vi "SVPO Analog Tacho Process (N Ch DBL WDT).vi"(0 "analog tacho signal":waveform(dbl)={"t0"=timestamp(0 s since 1904-01-01), "dt"=0.0, "Y"=[]}, 1 "AnalogTach States":T1, 5 "PPR":dbl, 7 "Thresh(V)":dbl, 9 "Slope":u16, 11 "hysteresis (0)":dbl format="%.2f", 12 "pulse width (2)":i32=2) -> (3 "AnalogTach States Out":T1, 4 "speed position info":T2)   [LabVIEW 2018, in "Measurement Channels.lvlib" / "Tachometer.lvclass"]
doc: "Locates tachometer pulse positions in analog tachometer signals. The data type you wire to the <B>analog tacho signal</B> input determines the polymorphic instance to use."
uses:
  Tachometer.lvclass
  <vilib>/addons/Sound and Vibration/Order Analysis/Misc/OAT Position Info.ctl
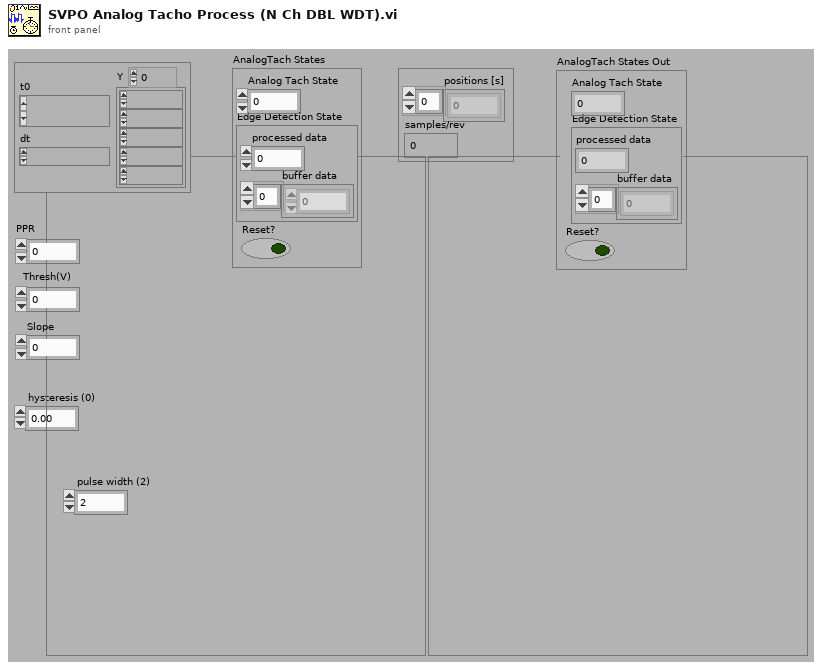
[diagram p1: front panel]
types:
  T1 = cluster{"Analog Tach State":dbl, "Edge Detection State":cluster{"processed data":dbl, "buffer data":dbl[]}, "Reset?":bool}
  T2 = typedef "OAT Position Info.ctl" = cluster{"positions [s]":dbl[], "samples/rev":dbl}
  T3 = cluster{"processed data":dbl, "buffer data":dbl[]}
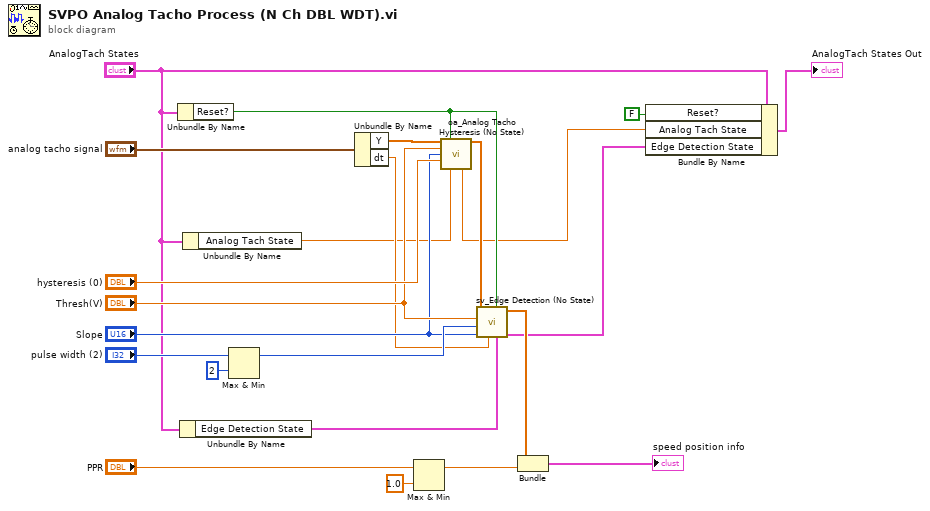
[diagram p0: block diagram]
diagram:
  n1 = Unbundle By Name("AnalogTach States") -> ("Reset?"=w6:bool)
  n2 = Unbundle By Name("AnalogTach States") -> ("Edge Detection State"=w7:T3)
  n3 = Unbundle By Name("AnalogTach States") -> ("Analog Tach State"=w8:dbl)
  n4 = Max & Min(x="pulse width (2)", y=2) -> (max(x,y)=w22:i32)  [unwired: 1 out]
  n5 = Unbundle By Name("analog tacho signal") -> ("Y"=w13:dbl[], "dt"=w11:dbl)
  n6 = Max & Min(x="PPR", y=1.0) -> (max(x,y)=w9:dbl)  [unwired: 1 out]
  n7 = call "oa_Analog Tacho Hysteresis (No State).vi"("input signal"=w13, "reset? (T)"=w6, "threshold (auto)"="Thresh(V)", "slope (Rising)"="Slope", "hysteresis(0)"="hysteresis (0)", "last value in"=w8) -> ("output signal"=w14:dbl[], "last value out"=w4:dbl)  [unwired: 7 in, 1 out]
  n8 = call "sv_Edge Detection (No State).vi"("state in"=w7, "reset? (True)"=w6, "dt"=w11, "slope (Rising)"="Slope", "pulse width (2)"=w22, "threshold (0.0)"="Thresh(V)", "x[n]"=w14) -> ("state out"=w3:T3, "pulse positions [s]"=w12:dbl[])  [unwired: 3 in]
  n9 = Bundle("pulse positions [s]"=w12, w9) -> (→"speed position info":cluster{"pulse positions [s]":dbl[], dbl})  [unwired: 1 in]
  n10 = Bundle By Name(cluster="AnalogTach States", "Reset?"=FALSE, "Analog Tach State"=w4, "Edge Detection State"=w3) -> (→"AnalogTach States Out":T1)
